vi "Get Distance.vi"(1 "refnum name":string="My Ultrasonic RefNum") -> (0 "distance":dbl)   [LabVIEW 2016]
doc: "DEPRECATED.\nGet the distance from an object using the ultrasonic sensor."
uses:
  <vilib>/ptbypt/NI_PtbyPt.lvlib
  <vilib>/Rock Robotics/WPI/Ultrasonic/WPI_UltrasonicRangeUnits.ctl
  <vilib>/Rock Robotics/WPI/Ultrasonic/WPI_SonarSRF04DigitalGetRange.vi
  <vilib>/Rock Robotics/WPI/Ultrasonic/WPI_SonarSRF04DigitalRefNum Registry Get.vi
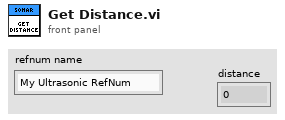
[diagram p1: front panel]
types:
  T1 = typedef "WPI_UltrasonicRangeUnits.ctl" = enum16{"inches", "mm"}
  T2 = typedef "WPI_UltrasonicDeviceRef.ctl" = cluster{"DevStatus":errorcluster, "Ping Channel":T3, "Echo Channel":T3, "CntIndex":T4}
  T3 = typedef "FPGA_DIOChannel.ctl" = enum8{"DIO 0", "DIO 1", "DIO 2", "DIO 3", "DIO 4", "DIO 5", "DIO 6", "DIO 7", "DIO 8", "DIO 9", "DIO MXP 0", "DIO MXP 1", "DIO MXP 2", "DIO MXP 3", "DIO MXP 4", "DIO MXP 5", "DIO MXP 6", "DIO MXP 7", "DIO MXP 8", "DIO MXP 9", "DIO MXP 10", "DIO MXP 11", "DIO MXP 12", "DIO MXP 13", "DIO MXP 14", "DIO MXP 15", "SPI Port CS1", "SPI Port CS2", "SPI Port CS3", "SPI Port MISO", "SPI Port MOSI", "Invalid"}
  T4 = typedef "FPGA_CounterCtrSystemIndex.ctl" = enum8{"Ctr 0", "Ctr 1", "Ctr 2", "Ctr 3", "Ctr 4", "Ctr 5", "Ctr 6", "Ctr 7", "Invalid"}
  T5 = typedef "WPI_UltrasonicDeviceRef.ctl" = cluster{"DevStatus":errorcluster, "Ping Digital Module":T6, "Echo Digital Module":T6, "Ping Channel":T7, "Echo Channel":T7, "CntIndex":T4}
  T6 = typedef "FPGA_TypedefDigitalModule.ctl" = enum16{"Digital Module 1", "Digital Module 2"}
  T7 = typedef "FPGA_DIOChannel.ctl" = enum8{"DIO 1", "DIO 2", "DIO 3", "DIO 4", "DIO 5", "DIO 6", "DIO 7", "DIO 8", "DIO 9", "DIO 10", "DIO 11", "DIO 12", "DIO 13", "DIO 14", "Invalid"}
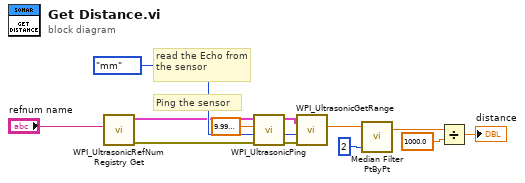
[diagram p0: block diagram]
diagram:
  # "read the Echo from the sensor"
  # "Ping the sensor"
  n1 = call-poly <vilib>:"WPI_UltrasonicRefNum Registry Get.vi"("refnum name"="refnum name") -> ("error out"=w3:errorcluster, "SonarSRF04DevRef"=w2:T2)  [unwired: 9 in]
  n2 = call <vilib>:"WPI_UltrasonicPing.vi"("error in (no error)"=w3, "pingtime (Sec)"=sgl 1e-05, "UltrasonicDevRef"=w2) -> ("error out"=w5:errorcluster, "UltrasonicDevRef"=w12:T5)  [unwired: 7 out]
  n3 = call-poly <vilib>:"WPI_UltrasonicGetRange.vi"(7:w12, "error in (no error)"=w5, 9:WPI_UltrasonicRangeUnits."mm" ("Range Units")) -> ("Distance"=w11:dbl)  [unwired: 6 in, 2 out]
  n4 = call <vilib>:"Median Filter PtByPt.vi"("rank"=2, "x"=w11) -> ("Filtered x"=w8:dbl)  [unwired: 2 in, 1 out]
  n5 = Divide(x=w8, y=1000.0) -> (x/y=→"distance":dbl)
